vi "GenerateCode.vi"(0 "XRef":T10, 1 "Terms":T7, 2 "Diagram":T6, 3 "State In":T1={"Type"=variant(bool FALSE)}) -> (14 "Generated Code?":T5, 15 "Reply":T3, 16 "Fatal Error Out":T2, 17 "State Out":T1={"Type"=variant(bool FALSE)})   [LabVIEW 2017, in "ReadTag.xnode"]
doc: "Read Tag XNode script that generates the block diagram code performing the tag read, and reports whether code was generated."
uses:
  ReadTag.xnode
  <vilib>/XNodeSupport/XNodeXNodeRef.ctl
  <vilib>/XNodeSupport/XNodeTermIDPairs.ctl
  <vilib>/XNodeSupport/XNodeTermIDPair.ctl
  <vilib>/XNodeSupport/XNodeTermRef.ctl
  <vilib>/XNodeSupport/XNodeString.ctl
  <vilib>/XNodeSupport/XNodeTopLevelDiagramRef.ctl
  State.ctl
  <vilib>/XNodeSupport/XNodeBool.ctl
  <vilib>/XNodeSupport/XNodeStringArray.ctl
  <vilib>/XNodeSupport/XNodeErrorCluster.ctl
  <vilib>/XNodeSupport/NI_XNodeSupport.lvlib
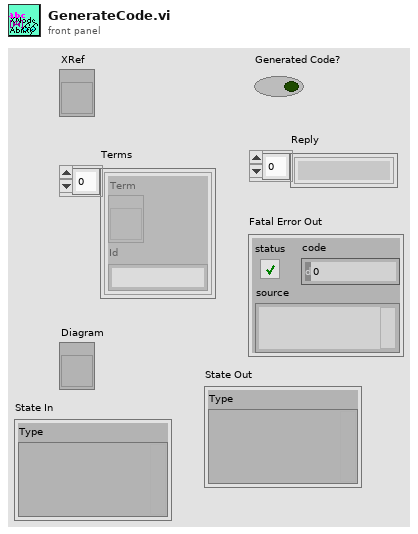
[diagram p1: front panel]
types:
  T1 = typedef "ReadTag.xnode/State.ctl" = cluster{"Type":variant}
  T2 = typedef "NI_XNodeSupport.lvlib/XNodeErrorCluster.ctl" = errorcluster
  T3 = typedef "NI_XNodeSupport.lvlib/XNodeStringArray.ctl" = T4[]
  T4 = typedef "NI_XNodeSupport.lvlib/XNodeString.ctl" = string
  T5 = typedef "NI_XNodeSupport.lvlib/XNodeBool.ctl" = bool
  T6 = typedef "NI_XNodeSupport.lvlib/XNodeTopLevelDiagramRef.ctl" = refnum<vi>
  T7 = typedef "NI_XNodeSupport.lvlib/XNodeTermIDPairs.ctl" = T8[]
  T8 = typedef "NI_XNodeSupport.lvlib/XNodeTermIDPair.ctl" = cluster{"Term":T9, "Id":T4}
  T9 = typedef "NI_XNodeSupport.lvlib/XNodeTermRef.ctl" = refnum<vi>
  T10 = typedef "NI_XNodeSupport.lvlib/XNodeXNodeRef.ctl" = refnum<vi>
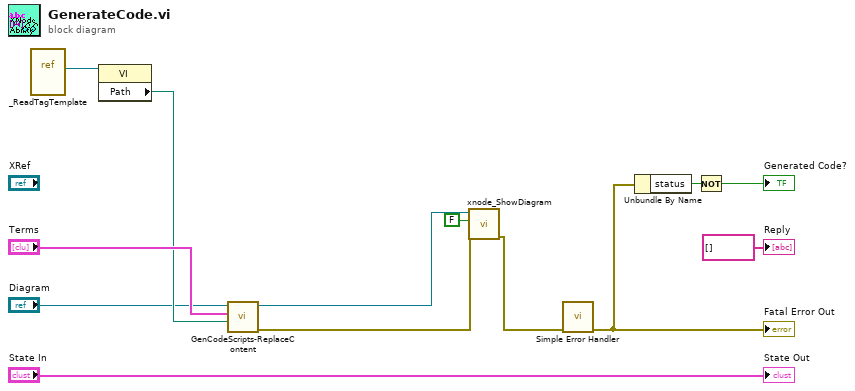
[diagram p0: block diagram]
diagram:
  n1 = vi-ref "_ReadTagTemplate.vi"() -> (w12:refnum<vi>)
  n2 = property class="VI"(reference=w12) -> ("Path"=w10:path)  [unwired: 1 in, 2 out]
  n3 = call "GenCodeScripts-ReplaceContent.vi"("template"=w10, "Terms"="Terms", "Diagram"="Diagram") -> ("error out"=w3:errorcluster, "Diagram out"=w5:T6)  [unwired: 6 in, 1 out]
  n4 = call "xnode_ShowDiagram.vi"("error in (no error)"=w3, "show?"=FALSE, "TopLevelDiagram in"=w5) -> ("error out"=w2:errorcluster)  [unwired: 7 in, 1 out]
  n5 = call <vilib>:"Simple Error Handler.vi"("error in (no error)"=w2) -> ("error out"=w7:errorcluster)  [unwired: 4 in, 4 out]
  "Fatal Error Out" <- w7
  n6 = Unbundle By Name(w7) -> ("status"=w8:bool)
  n7 = Not(x=w8) -> (.not. x?=→"Generated Code?":bool)
  "Reply" <- T3 [] ("Reply")
  "State Out" <- "State In"
